vi "WaitForWinding.vi"(8 "Error In":errorcluster, 11 "AutoData":T1) -> (0 "Error Out":errorcluster, 3 "AutoData out":T1)   [LabVIEW 2019, in "AutoMode.lvlib"]
uses:
  AutoMode.lvlib
  Cluster - AutoModeData.ctl
  MainController/Cluster - TestSettings.ctl
  MainController/Cluster - HardwareConfiguration.ctl
  MainController/Cluster - TestResults.ctl
  Cluster - AutoModeMessage.ctl
  Enum - AutoModeState.ctl
  MainController/Cluster - MainControllerMessage.ctl
  MainController/Enum - MainState.ctl
  Mark10 API/Mark 10 TSTM-DC.lvlib
  Timer/Timer.lvlib
  Mark10 API/ReadTravelAndForce.vi
  MainController/MainController.lvlib
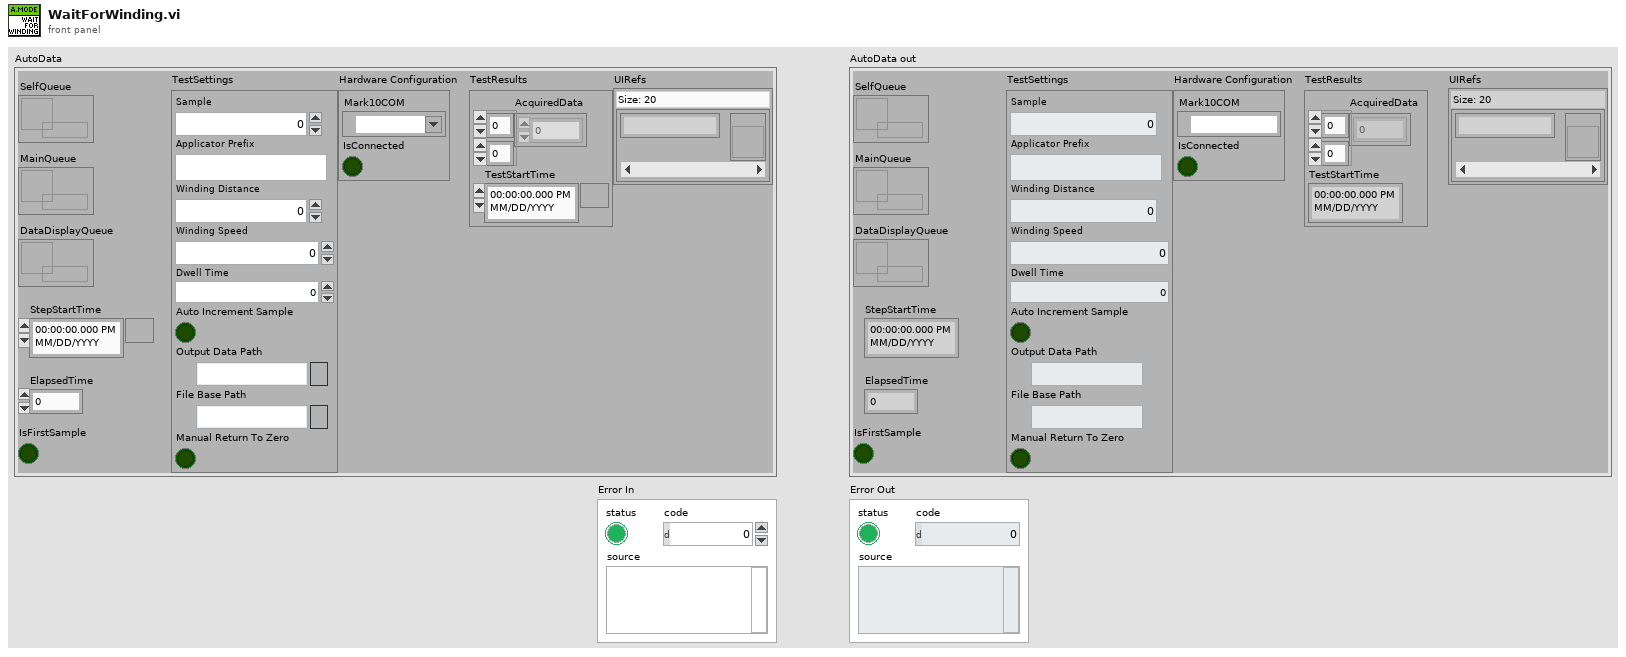
[diagram p1: front panel]
types:
  T1 = typedef "AutoMode.lvlib/Cluster - AutoModeData.ctl" = cluster{"DataDisplayQueue":refnum<queue>, "StepStartTime":timestamp, "TestSettings":T2, "Hardware Configuration":T3, "TestResults":T4, "ElapsedTime":dbl, "IsFirstSample":bool, "UIRefs":map{string, refnum<vi>}, "SelfQueue":refnum<queue>, "MainQueue":refnum<queue>}
  T2 = typedef "MainController.lvlib/Cluster - TestSettings.ctl" = cluster{"Sample":u32, "Applicator Prefix":string, "Winding Distance":dbl, "Winding Speed":dbl, "Dwell Time":dbl, "Auto Increment Sample":bool, "Output Data Path":path, "File Base Path":path, "Manual Return To Zero":bool}
  T3 = typedef "MainController.lvlib/Cluster - HardwareConfiguration.ctl" = cluster{"Mark10COM":refnum<visa-resource-name>, "IsConnected":bool}
  T4 = typedef "MainController.lvlib/Cluster - TestResults.ctl" = cluster{"AcquiredData":dbl[][], "TestStartTime":timestamp}
  T5 = typedef "AutoMode.lvlib/Enum - AutoModeState.ctl" = enum16{"Initialize", "Idle", "UpdateConfig", "UpdateHWConfig", "BroadcastSettings", "Start", "CheckValidReportPath", "Winding", "WaitForWinding", "Unwind", "WaitForUnwind", "Stop", "Abort", "WriteDataToFile", "EventTriggered", "GenerateFilePath", "ZeroPosition", "GotoZero", "Error", "Exit"}
  T6 = typedef "Mark 10 TSTM-DC.lvlib/Cluster - FeedbackData.ctl" = cluster{"Angle":dbl, "Torque":dbl, "Work":dbl}
  T7 = cluster{"number: 0 to 1":dbl, "number: 0 to 1":dbl, "number: 0 to 1":dbl}
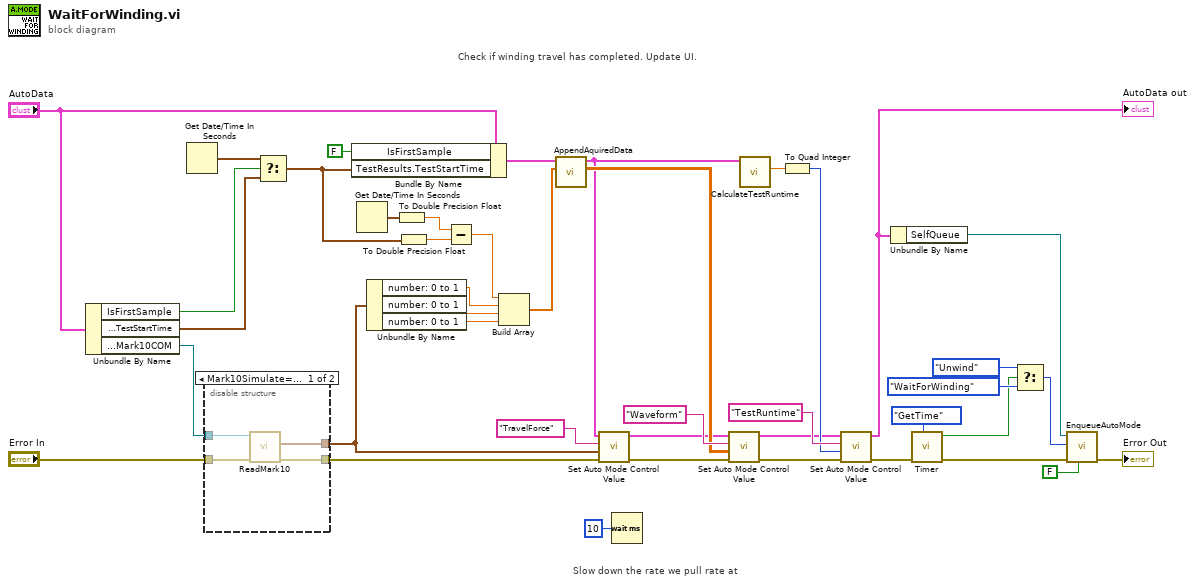
[diagram p0: block diagram]
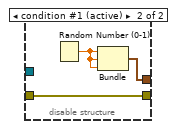
[diagram p2: hidden frame]
diagram:
  # "Check if winding travel has completed. Update UI."
  # "Slow down the rate we pull rate at"
  n1 = Unbundle By Name("AutoData") -> ("IsFirstSample"=w21:bool, "TestResults.TestStartTime"=w25:timestamp, "Hardware Configuration.Mark10COM"=w42:refnum<visa-resource-name>)
  n2 = Get Date/Time In Seconds() -> (seconds since 1Jan1904=w26:timestamp)
  n3 = disable-structure shown="Mark10Simulate==False, Default" {
    disable-tunnel: w42 -> [w46 _]
    disable-tunnel: "Error In" -> [w45 w49]
    disable-tunnel: [w44 w49] -> w10
    disable-tunnel: [w43 w47] -> w9
    frame condition #0 {
      n4 = call-poly "ReadMark10.vi"("error in"=w45, "VISA resource name"=w46) -> ("error out"=w44:errorcluster, "FeedbackData"=w43:T6)  [unwired: 7 in, 1 out]
    }
    frame condition #1 (active) {
      n5 = Random Number (0-1)() -> (number: 0 to 1=w48:dbl)
      n6 = Bundle("number: 0 to 1"=w48, "number: 0 to 1"=w48, "number: 0 to 1"=w48) -> (w47:T7)  [unwired: 1 in]
    }
  }
  n7 = Select(t=w26, s=w21, f=w25) -> (s? t:f=w23:timestamp)
  n8 = Bundle By Name(cluster="AutoData", "IsFirstSample"=FALSE, "TestResults.TestStartTime"=w23) -> (w24:T1)
  n9 = Get Date/Time In Seconds() -> (seconds since 1Jan1904=w38:timestamp)
  n10 = Unbundle By Name(w9) -> ("number: 0 to 1"=w39:dbl, "number: 0 to 1"=w40:dbl, "number: 0 to 1"=w41:dbl)
  n11 = To Double Precision Float(number=w38) -> (double precision float=w32:dbl)
  n12 = To Double Precision Float(number=w23) -> (double precision float=w31:dbl)
  n13 = Subtract(x=w32, y=w31) -> (x-y=w30:dbl)
  n14 = Build Array(w30, w39, w40, w41) -> (w36:dbl[])
  n15 = call "AppendAquiredData.vi"("Array"=w36, "CycleTestData in"=w24) -> ("TestData"=w14:dbl[][], "CycleTestData out"=w7:T1)  [unwired: 8 in]
  n16 = call "Set Auto Mode Control Value.vi"("Error In"=w10, "Value"=w9, "key"="TravelForce", "AutoData"=w7) -> ("Error Out"=w11:errorcluster, "AutoData out"=w8:T1)  [unwired: 6 in]
  n17 = Wait (ms)(milliseconds to wait=u32 10) -> ()  [unwired: 1 out]
  n18 = call "Set Auto Mode Control Value.vi"("Error In"=w11, "Value"=w14, "key"="Waveform", "AutoData"=w8) -> ("Error Out"=w13:errorcluster, "AutoData out"=w15:T1)  [unwired: 6 in]
  n19 = call "CalculateTestRuntime.vi"("AutoData"=w7) -> ("ElapsedTime"=w29:dbl)  [unwired: 10 in]
  n20 = To Quad Integer(1:w29) -> (0:w17:i64)
  n21 = call "Set Auto Mode Control Value.vi"("Error In"=w13, "Value"=w17, "key"="TestRuntime", "AutoData"=w15) -> ("Error Out"=w5:errorcluster, "AutoData out"=w3:T1)  [unwired: 6 in]
  "AutoData out" <- w3
  n22 = Unbundle By Name(w3) -> ("SelfQueue"=w2:refnum<queue>)
  n23 = call "Timer.vi"("TimerState"=enum16{"Reset", "Start", "GetTime", "Stop"}."GetTime", "Error In"=w5) -> ("Error Out"=w4:errorcluster, "IsTimeElapsed"=w27:bool)  [unwired: 8 in]
  n24 = Select(t=Enum_-_AutoModeState."Unwind" ("CycleTestState"), s=w27, f=Enum_-_AutoModeState."WaitForWinding" ("CycleTestState")) -> (s? t:f=w33:T5)
  n25 = call "EnqueueAutoMode.vi"("Priority Message"=FALSE, "error in (no error)"=w4, "AutoState"=w33, "Queue in"=w2) -> ("error out"=→"Error Out":errorcluster)  [unwired: 6 in, 1 out]
